vi "SPARK Get Status 8.vi"(8 "error in (no error)":errorcluster, 11 "MotorControlDeviceRef in":T3={"DeviceStatus"={"status"=FALSE, "code"=0, "source"=""}, "Type"=enum."PWM", "PWM"={"PWM Channel"=enum."Invalid", "DeadBand"={"Name"="", "maxPositivePwm"=0, "minPositivePwm"=0, "centerPwm"=0, "maxNegativePwm"=0, "minNegativePwm"=0, "angularRange"=0}}, "CAN"={"Device Number"=0, "SetOutput VI Ref"=variant, "GetOutput VI Ref"=variant, "Enable VI Ref"=variant, "Disable VI Ref"=variant, "Data"=variant}, "Invert"=FALSE, "DIO PWM"={"PWM \"Enable\" Channel"=enum."Invalid", "DIOChannel"=enum."Invalid", "PWM Rate"=0.0}}) -> (0 "error out":errorcluster, 2 "Status 8 Frame":T1 {"Selected PID Slot" items=["Slot 0", "Slot 1", "Slot 2", "Slot 3"]}, 3 "MotorControlDeviceRef out":T3={"DeviceStatus"={"status"=FALSE, "code"=0, "source"=""}, "Type"=enum."PWM", "PWM"={"PWM Channel"=enum."Invalid", "DeadBand"={"Name"="", "maxPositivePwm"=0, "minPositivePwm"=0, "centerPwm"=0, "maxNegativePwm"=0, "minNegativePwm"=0, "angularRange"=0}}, "CAN"={"Device Number"=0, "SetOutput VI Ref"=variant, "GetOutput VI Ref"=variant, "Enable VI Ref"=variant, "Disable VI Ref"=variant, "Data"=variant}, "Invert"=FALSE, "DIO PWM"={"PWM \"Enable\" Channel"=enum."Invalid", "DIOChannel"=enum."Invalid", "PWM Rate"=0.0}})   [LabVIEW 2023]
uses:
  <vilib>/Rock Robotics/WPI/MotorControl/WPI_MotorControlDeviceRef.ctl
  <vilib>/Rock Robotics/WPI/MotorControl/WPI_MotorControlType.ctl
  <vilib>/Rock Robotics/SystemInterfaces/DIO/FPGA_DIOPWMChannel.ctl
  <vilib>/Rock Robotics/WPI/PWM/WPI_PWMDeadband.ctl
  <vilib>/Rock Robotics/SystemInterfaces/DIO/FPGA_DIOChannel.ctl
  Typedef/SPARK Status 8 Frame.ctl
  Typedef/SPARK Closed Loop Slot.ctl
  Typedef/Spark MAX Variant Data.ctl
  Typedef/SPARK Model.ctl
  Typedef/SPARK Periodic Status.ctl
  Typedef/SPARK CAN Arb ID.ctl
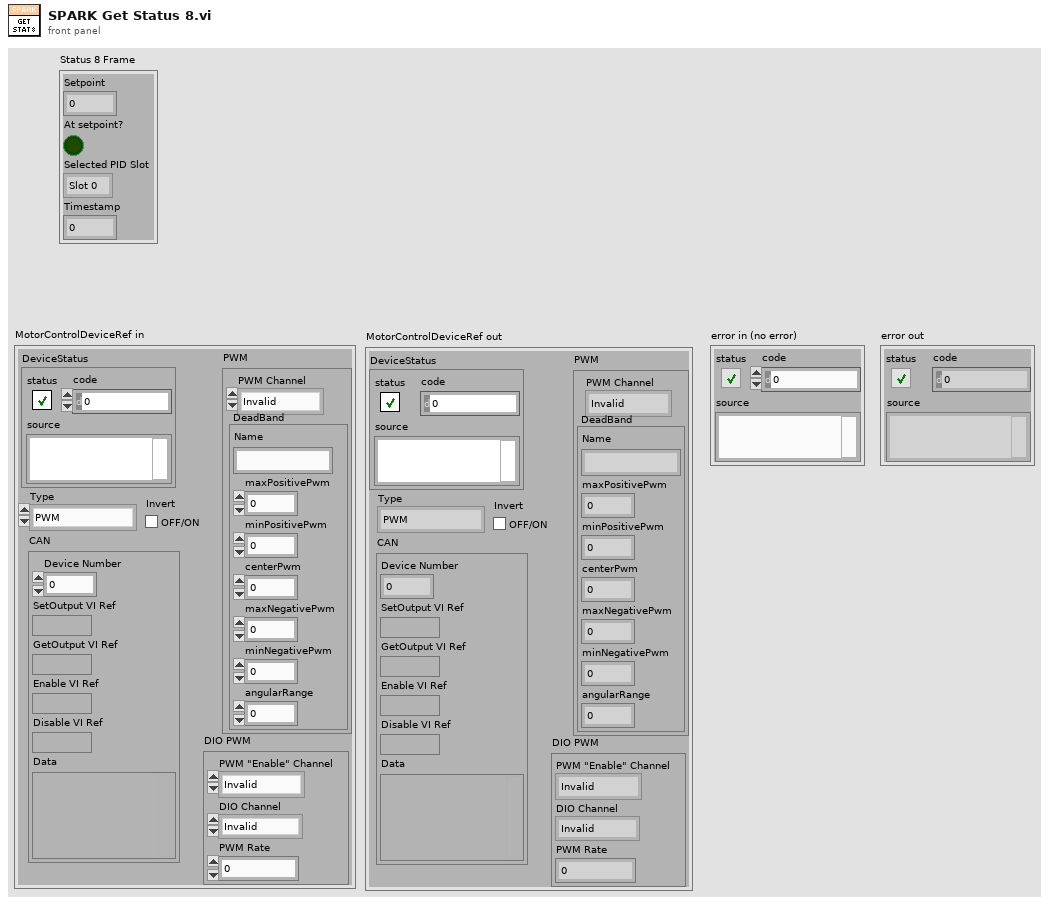
[diagram p1: front panel]
types:
  T1 = typedef "SPARK Status 8 Frame.ctl" = cluster{"Setpoint":sgl, "At setpoint?":bool, "Selected PID Slot":T2, "Timestamp":u32}
  T2 = typedef "SPARK Closed Loop Slot.ctl" = u16
  T3 = typedef "WPI_MotorControlDeviceRef.ctl" = cluster{"DeviceStatus":errorcluster, "Type":T4, "PWM":cluster{"PWM Channel":T5, "DeadBand":T6}, "CAN":cluster{"Device Number":u8, "SetOutput VI Ref":variant, "GetOutput VI Ref":variant, "Enable VI Ref":variant, "Disable VI Ref":variant, "Data":variant}, "Invert":bool, "DIO PWM":cluster{"PWM \"Enable\" Channel":T5, "DIOChannel":T7, "PWM Rate":dbl}}
  T4 = typedef "WPI_MotorControlType.ctl" = enum16{"PWM", "CAN", "DIO PWM"}
  T5 = typedef "FPGA_DIOPWMChannel.ctl" = enum8{"PWM 0", "PWM 1", "PWM 2", "PWM 3", "PWM 4", "PWM 5", "PWM 6", "PWM 7", "PWM 8", "PWM 9", "PWM MXP 0", "PWM MXP 1", "PWM MXP 2", "PWM MXP 3", "PWM MXP 4", "PWM MXP 5", "PWM MXP 6", "PWM MXP 7", "PWM MXP 8", "PWM MXP 9", "Invalid"}
  T6 = typedef "WPI_PWMDeadband.ctl" = cluster{"Name":string, "maxPositivePwm":i32, "minPositivePwm":i32, "centerPwm":i32, "maxNegativePwm":i32, "minNegativePwm":i32, "angularRange":u16}
  T7 = typedef "FPGA_DIOChannel.ctl" = enum8{"DIO 0", "DIO 1", "DIO 2", "DIO 3", "DIO 4", "DIO 5", "DIO 6", "DIO 7", "DIO 8", "DIO 9", "DIO MXP 0", "DIO MXP 1", "DIO MXP 2", "DIO MXP 3", "DIO MXP 4", "DIO MXP 5", "DIO MXP 6", "DIO MXP 7", "DIO MXP 8", "DIO MXP 9", "DIO MXP 10", "DIO MXP 11", "DIO MXP 12", "DIO MXP 13", "DIO MXP 14", "DIO MXP 15", "SPI Port CS1", "SPI Port CS2", "SPI Port CS3", "SPI Port MISO", "SPI Port MOSI", "Invalid"}
  T8 = typedef "SPARK CAN Arb ID.ctl" = u32
  T9 = typedef "SPARK Periodic Status.ctl" = enum16{"Periodic Status 0", "Periodic Status 1", "Periodic Status 2", "Periodic Status 3", "Periodic Status 4", "Periodic Status 5", "Periodic Status 6", "Periodic Status 7", "Periodic Status 8", "Periodic Status 9"}
  T10 = typedef "Spark MAX Variant Data.ctl" = cluster{"Ext ID":u32, "CAN Timeout":u32, "Inverted No WPILib":bool, "Has Configured Limit Sw":bool, "Has Configured Alt Encoder":bool, "SPARK Model":T11, "CAN Max Retries":u32, "CAN Timeout (ms)":u32, "Status 0 Period (ms)":u32, "Status 1 Period (ms)":u32, "Status 2 Period (ms)":u32, "Status 3 Period (ms)":u32, "Status 4 Period (ms)":u32, "Status 5 Period (ms)":u32, "Status 6 Period (ms)":u32, "Status 7 Period (ms)":u32, "Status 8 Period (ms)":u32, "Status 9 Period (ms)":u32, "Status Frame Timeout (ms)":u32}
  T11 = typedef "SPARK Model.ctl" = enum16{"SPARK MAX", "SPARK Flex", "Unknown"}
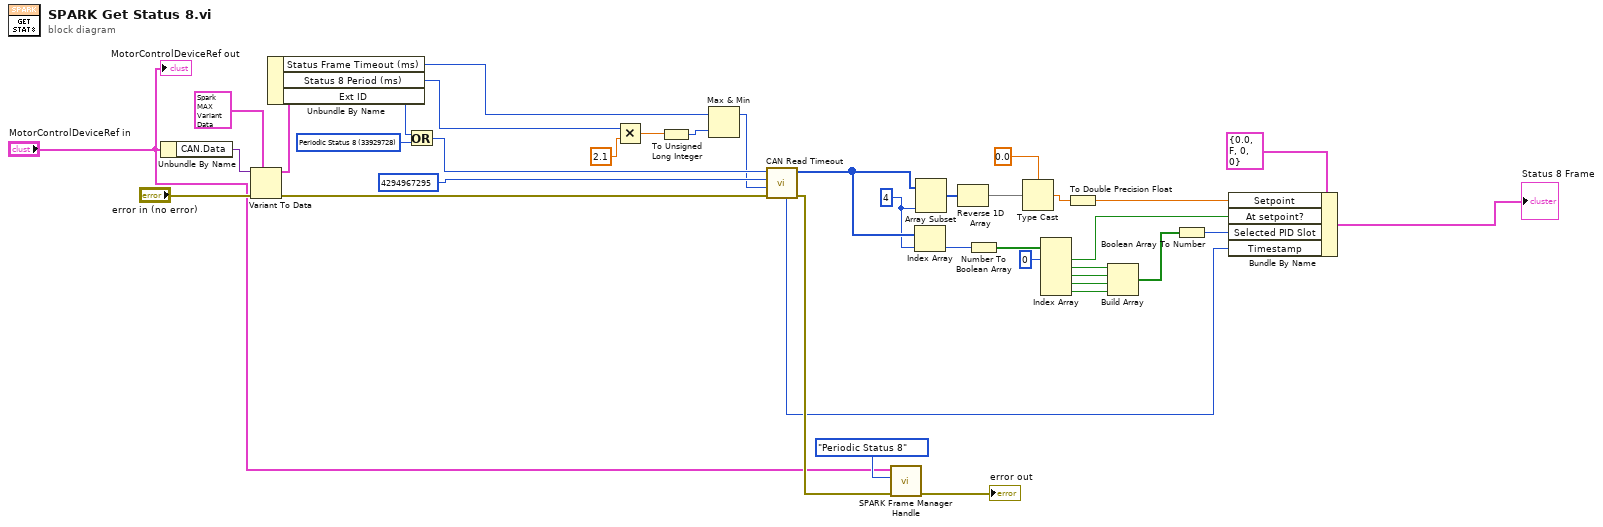
[diagram p0: block diagram]
diagram:
  w15 = T8 33929728 items=["Broadcast Disable"=0, "Broadcast System Halt"=64, "Broadcast System Reset"=128, "Broadcast Device Assign"=192, "Broadcast Heartbeat"=320, "Broadcast Firmware Version"=512, "Broadcast Enumerate"=576, "Broadcast System Resume"=640, "Velocity Setpoint"=33882112, "Duty Cycle Setpoint"=33882240, "Smart Velocity Setpoint"=33882304, "Position Setpoint"=33882368, "Voltage Setpoint"=33882432, "Current Setpoint"=33882496, "Smart Motion Setpoint"=33882560, "MAXMotion Position Setpoint"=33882624, "MAXMotion Velocity Setpoint"=33882688, "Periodic Status 0"=33929216, "Periodic Status 1"=33929280, "Periodic Status 2"=33929344, "Periodic Status 3"=33929408, "Periodic Status 4"=33929472, "Periodic Status 5"=33929536, "Periodic Status 6"=33929600, "Periodic Status 7"=33929664, "Periodic Status 8"=33929728, "Set Statuses Enabled"=33883136, "Set Statuses Enabled Response"=33883200, "DRV Status"=33888896, "Clear Faults"=33889152, "Parameter Write"=33896448, "Parameter Write Response"=33896512, "Parameter Double Read Start (RTR)"=33897472, "Persist Parameters"=33947584, "Persist Parameters Response"=33883392, "Reset Parameters"=33883456, "Reset Parameters Response"=33883520, "Set Follower Mode"=33889472, "Nack"=33890304, "Ack"=33890368, "Broadcast (not a command)"=33891328, "Heartbeat"=33891456, "Sync"=33891520, "IDQuery"=33891584, "IDAssign"=33891648, "Get Motor Interface (RTR)"=33894720, "Get Firmware Version (RTR)"=33891840, "REV Enumerate"=33891904, "Legacy/USB Heartbeat"=33891968, "roboRIO Lock"=33892032, "SWDL Data"=33892096, "SWDL Checksum"=33892160, "SWDL Retransmit"=33892224, "Set Primary Encoder Position"=33892352, "Set I Accum"=33892480, "Set Alt or Ext Encoder Position"=33892608, "Non-roboRIO Broadcast (not a command)"=33893376, "non-RIO Lock"=33893440, "Start Follower Mode"=33913856, "Start Follower Mode Response"=33913920, "Stop Follower Mode"=33913984, "Stop Follower Mode Response"=33914048, "non-RIO Heartbeat"=33893504] ("SPARK Arb ID")
  w11 = 4 ("length")
  n1 = Unbundle By Name("MotorControlDeviceRef in") -> ("CAN.Data"=w39:variant)
  n2 = Variant To Data(error in="error in (no error)", type=T10 {"Ext ID"=0, "CAN Timeout"=0, "Inverted No WPILib"=FALSE, "Has Configured Limit Sw"=FALSE, "Has Configured Alt Encoder"=FALSE, "SPARK Model"=enum."Unknown", "CAN Max Retries"=5, "CAN Timeout (ms)"=20, "Status 0 Period (ms)"=10, "Status 1 Period (ms)"=250, "Status 2 Period (ms)"=20, "Status 3 Period (ms)"=20, "Status 4 Period (ms)"=20, "Status 5 Period (ms)"=20, "Status 6 Period (ms)"=20, "Status 7 Period (ms)"=20, "Status 8 Period (ms)"=20, "Status 9 Period (ms)"=20, "Status Frame Timeout (ms)"=500} ("SPARK MAX Device Ref"), Variant=w39) -> (data=w36:T10, error out=w32:errorcluster)
  n3 = Unbundle By Name(w36) -> ("Status Frame Timeout (ms)"=w16:u32, "Status 8 Period (ms)"=w17:u32, "Ext ID"=w35:u32)
  n4 = Or(x=w35, y=w15) -> (x .or. y?=w34:T8)
  n5 = Multiply(x=w17, y=2.1) -> (x*y=w20:dbl)
  n6 = To Unsigned Long Integer(number=w20) -> (unsigned 32bit integer=w19:u32)
  n7 = Max & Min(x=w16, y=w19) -> (max(x,y)=w18:u32)  [unwired: 1 out]
  n8 = call "CAN Read Timeout.vi"("error in (no error)"=w32, "Timeout (ms)"=w18, "Message ID Mask"=u32 4294967295, "Message ID"=w34) -> ("error out"=w26:errorcluster, "data"=w12:u8[], "timestamp"=w23:u32)  [unwired: 5 in]
  n9 = call "SPARK Frame Manager Handle.vi"("error in (no error)"=w26, "Periodic Status"=SPARK_Periodic_Status."Periodic Status 8", "MotorControlDeviceRef"="MotorControlDeviceRef in") -> ("error out"=→"error out":errorcluster)  [unwired: 8 in]
  n10 = Index Array(array=w12, index=w11) -> (element=w10:u8)
  n11 = Array Subset(array=w12, length=w11) -> (w31:u8[])  [unwired: 1 in]
  n12 = Reverse 1D Array(array=w31) -> (reversed array=w30:u8[])
  n13 = Number To Boolean Array(number=w10) -> (Boolean array=w9:bool[])
  n14 = Type Cast(type=sgl 0.0, x=w30) -> (*(type *) &x=w28:sgl)
  n15 = Index Array(array=w9, index #1=0 ("index")) -> (element #1=w8:bool, element #2=w6:bool, element #3=w5:bool, element #4=w4:bool, element #5=w3:bool)  [unwired: 4 in]
  n16 = To Double Precision Float(number=w28) -> (double precision float=w27:dbl)
  n17 = Build Array(w6, w5, w4, w3) -> (w2:bool[])
  n18 = Boolean Array To Number(Boolean array=w2) -> (number=w1:u32)
  n19 = Bundle By Name(cluster=T1 {"Setpoint"=0.0, "At setpoint?"=FALSE, "Selected PID Slot"=0, "Timestamp"=0} ("SPARK Status 8"), "Setpoint"=w27, "At setpoint?"=w8, "Selected PID Slot"=w1, "Timestamp"=w23) -> (→"Status 8 Frame":T1)
  "MotorControlDeviceRef out" <- "MotorControlDeviceRef in"
